vi "Find highest intensity filter position.vi"(8 "error in":errorcluster, 10 "No of points":i32=2, 11 "VISA resource name out":refnum<visa-resource-name>) -> (0 "error out":errorcluster, 2 "Average time step (s)":sgl, 3 "Angle to no filter (deg.)":sgl)   [LabVIEW 2016]
uses:
  C:/Program Files (x86)/National Instruments/LabVIEW 2016/instr.lib/keithley_24xx/Keithley 24XX/Public/Data/Read (Multiple Points).vi
  C:/Program Files (x86)/National Instruments/LabVIEW 2016/instr.lib/keithley_24xx/Keithley 24XX/Keithley 24XX.lvlib
panel:
  out "x*y":dbl
  out "element":dbl
  out "Measurement times (s)":sgl[](array[numeric])
  out "J-t":sgl[][](array[numeric]) format="%#_11g"
  out "J-t":cluster{dbl[], "Current":sgl[]}(graph)
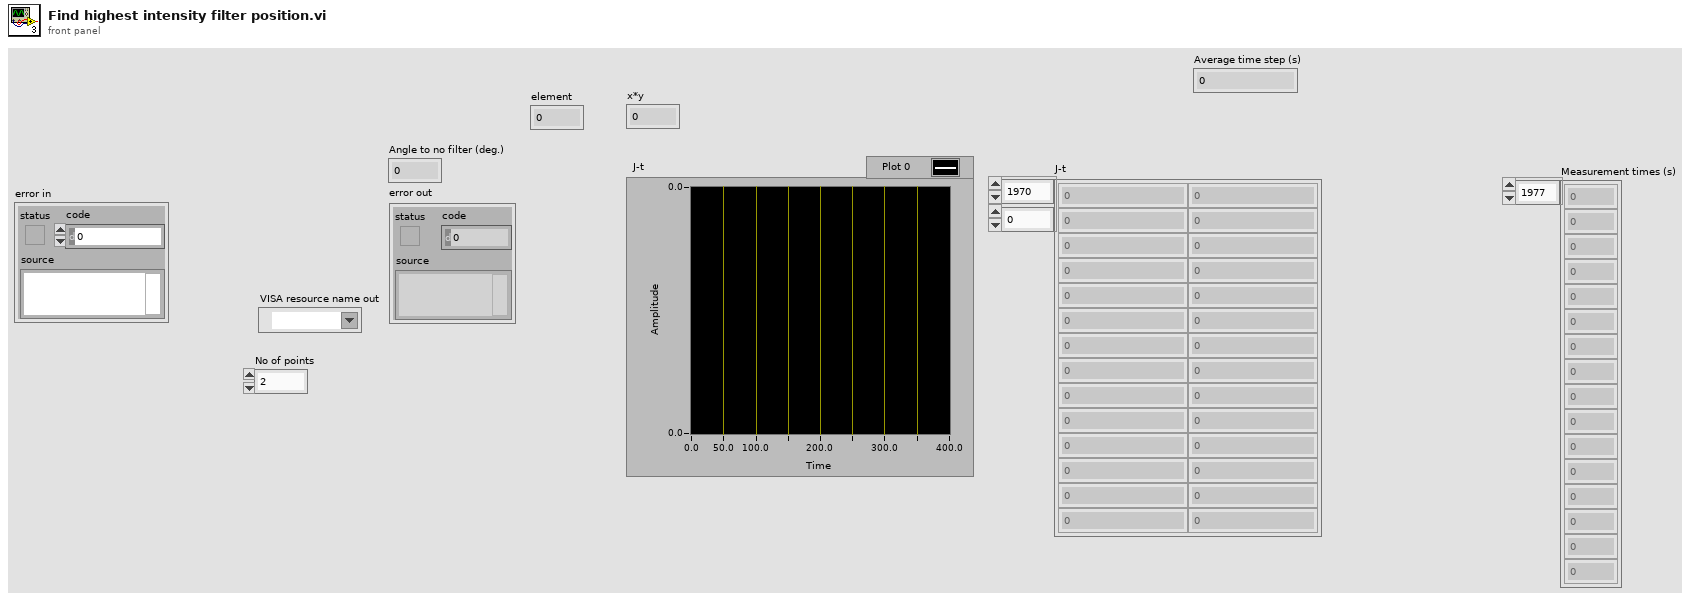
[diagram p1: front panel]
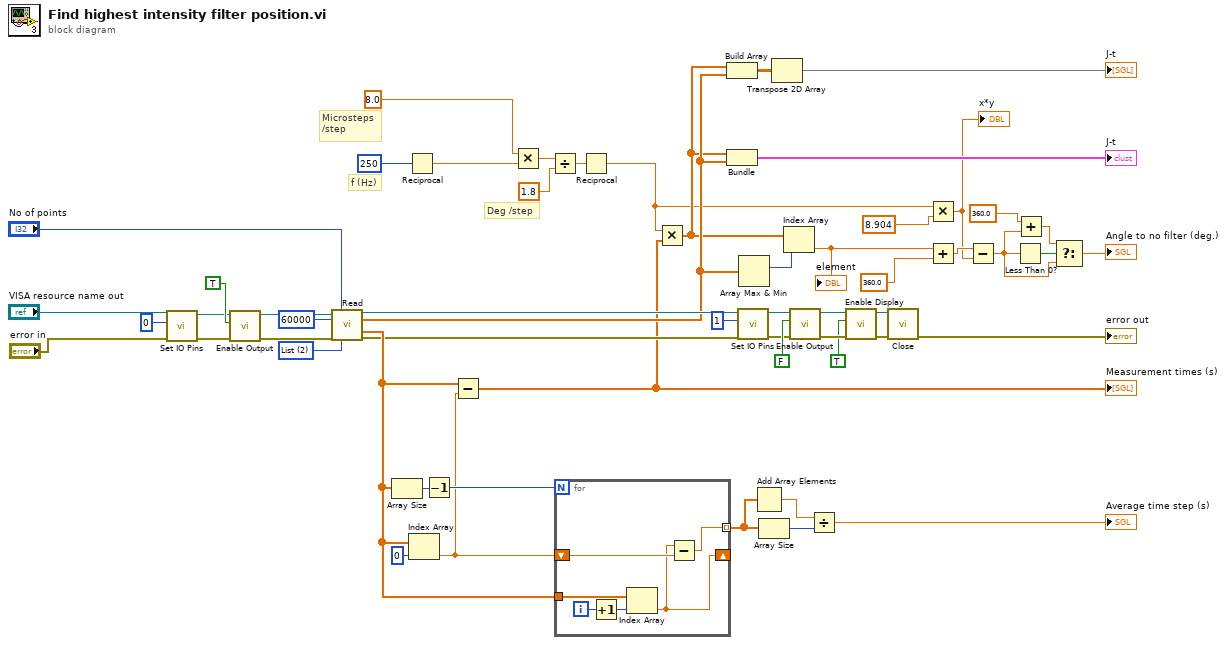
[diagram p0: block diagram]
diagram:
  w40 = u16 2 items=["Fixed", "Sweep", "List"] ("Output Mode (0: Fixed)")
  # "f (Hz)"
  # "Microsteps\n/step"
  # "Deg /step"
  n1 = call "Set IO Pins.vi"("error in (no error)"="error in", "Output Pattern (0)"=0, "VISA resource name"="VISA resource name out") -> ("error out"=w28:errorcluster, "VISA resource name out"=w30:refnum<visa-resource-name>)  [unwired: 7 in]
  n2 = call "Enable Output.vi"("error in (no error)"=w28, "Enable Output (T: Enable)"=TRUE ("Output (Off)"), "VISA resource name"=w30) -> ("error out"=w33:errorcluster, "VISA resource name out"=w34:refnum<visa-resource-name>)  [unwired: 7 in]
  n3 = call-poly "Read.vi"("VISA resource name"=w34, "Sample Count (1)"="No of points", "Timeout (10000 ms)"=60000, "error in (no error)"=w33, "Output Mode (0: Fixed)"=w40) -> ("VISA resource name out"=w38:refnum<visa-resource-name>, "Current"=w27:sgl[], "Timestamp"=w37:sgl[], "error out"=w36:errorcluster)  [unwired: 4 in, 3 out]
  n4 = Array Size(array=w37) -> (size(s)=w43:i32)
  n5 = Reciprocal(x=u32 250 ("Frequency (Hz)")) -> (1/x=w20:dbl)
  n6 = Index Array(array=w37, index=0) -> (element=w42:sgl)
  n7 = Decrement(x=w43) -> (x-1=w44:i32)
  n8 = Subtract(x=w37, y=w42) -> (x-y=w7:sgl[])
  "Measurement times (s)" <- w7
  n9 = Multiply(x=8.0 ("y"), y=w20) -> (x*y=w18:dbl)
  n10 = Divide(x=w18, y=1.8) -> (x/y=w16:dbl)
  n11 = for {
    N: w44 -> [_]
    tunnel: w37 -> [w60]
    shift-right: [w58] -> _
    shift-left: w42 -> [w59]
    tunnel: [w57] -> w51 mode=indexing
    i -> [w62]
    n12 = Increment(x=w62) -> (x+1=w61:i32)
    n13 = Index Array(array=w60, index=w61) -> (element=w58:sgl)
    n14 = Subtract(x=w58, y=w59) -> (x-y=w57:sgl)
  }
  n15 = Reciprocal(x=w16) -> (1/x=w12:dbl)
  n16 = Multiply(x=w12, y=w7) -> (x*y=w15:dbl[])
  n17 = Build Array(w15, w27) -> (w46:dbl[][])
  n18 = Bundle(w15, "Current"=w27) -> (→"J-t":cluster{dbl[], "Current":sgl[]})  [unwired: 1 in]
  n19 = call "Set IO Pins.vi"("error in (no error)"=w36, "Output Pattern (0)"=1, "VISA resource name"=w38) -> ("error out"=w53:errorcluster, "VISA resource name out"=w55:refnum<visa-resource-name>)  [unwired: 7 in]
  n20 = Array Max & Min(array=w27) -> (max index (indices)=w41:i32)  [unwired: 3 out]
  n21 = Add Array Elements(numeric array=w51) -> (sum=w49:sgl)
  n22 = Array Size(array=w51) -> (size(s)=w50:i32)
  n23 = Transpose 2D Array(2D array=w46) -> (transposed array=→"J-t":dbl[][])
  n24 = Index Array(array=w15, index=w41) -> (element=w5:dbl)
  "element" <- w5
  n25 = call "Enable Output.vi"("error in (no error)"=w53, "Enable Output (T: Enable)"=FALSE ("Output (Off)"), "VISA resource name"=w55) -> ("error out"=w24:errorcluster, "VISA resource name out"=w26:refnum<visa-resource-name>)  [unwired: 7 in]
  n26 = Divide(x=w49, y=w50) -> (x/y=→"Average time step (s)":sgl)
  n27 = call "Enable Display.vi"("error in (no error)"=w24, "Enable Display (T: Enable)"=TRUE ("Enable Output (T: Enable)"), "VISA resource name"=w26) -> ("error out"=w23:errorcluster, "VISA resource name out"=w25:refnum<visa-resource-name>)  [unwired: 7 in]
  n28 = call "Close.vi"("error in (no error)"=w23, "VISA resource name"=w25) -> ("error out"=→"error out":errorcluster)  [unwired: 9 in]
  n29 = Multiply(x=w12, y=8.904) -> (x*y=w1:dbl)
  "x*y" <- w1
  n30 = Add(x=w5, y=360.0 ("x")) -> (x+y=w2:dbl)
  n31 = Subtract(x=w2, y=w1) -> (x-y=w3:dbl)
  n32 = Less Than 0?(x=w3) -> (x < 0?=w11:bool)
  n33 = Add(x=360.0, y=w3) -> (x+y=w9:dbl)
  n34 = Select(t=w9, s=w11, f=w3) -> (s? t:f=→"Angle to no filter (deg.)":dbl)
